vi "Ohm.vi"() -> (3 "Numeric":dbl)   [LabVIEW 2012]
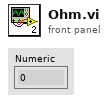
[diagram p1: front panel]
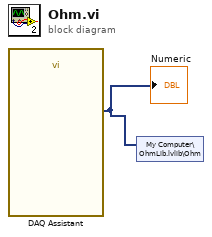
[diagram p0: block diagram]
diagram:
  n1 = call "DAQ Assistant"() -> ("data"=w1:dynamicdata)  [unwired: 17 in, 2 out]
  "Numeric" <- w1
  n2 = shared-variable "My Computer\\OhmLib.lvlib\\Ohm"(w1) -> ()  [unwired: 1 in, 1 out]
